vi "Tracepoint_LoadStaleFiles.vi"(8 "error in (no error)":errorcluster, 10 "file paths":path[](array[path]), 11 "Qbus in":refnum<class "Qbus.lvclass">) -> (0 "error out":errorcluster)   [LabVIEW 2017, in "FileManager.lvlib"]
uses:
  <vilib>/addons/InsightCM/Devices/Shared/Common/FileManager/FileManager.lvlib
  <vilib>/addons/Qbus/Qbus.lvclass
  <vilib>/addons/TraceLogger/TraceLogger.lvlib
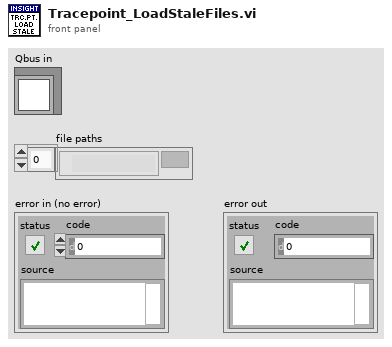
[diagram p1: front panel]
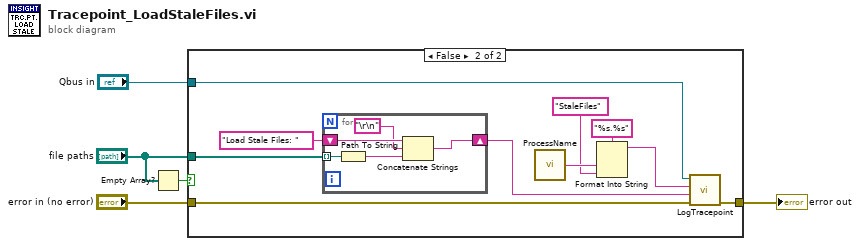
[diagram p0: block diagram]
diagram:
  n1 = Empty Array?(array="file paths") -> (empty?=w3:bool)
  n2 = case shown="False" w3 {
    tunnel: "file paths" -> [_ w9]
    tunnel: "error in (no error)" -> [w6 w12]
    tunnel: [w6 w11] -> w4
    tunnel: "Qbus in" -> [_ w10]
    frame True {
    }
    frame False {
      n3 = for {
        tunnel: w9 -> [w19] mode=indexing
        shift-right: [w21] -> w8
        shift-left: "Load Stale Files: " -> [w20]
        n4 = Path To String(path=w19) -> (string=w18:string)
        n5 = Concatenate Strings(w20, "\r\n", w18) -> (w21:string)
      }
      n6 = call <vilib>:"ProcessName.vi"() -> ("process name"=w16:string)  [unwired: 5 in]
      n7 = Format Into String(format string="%s.%s", w16, "StaleFiles" ("tracepoint")) -> (resulting string=w13:string)  [unwired: 2 in, 1 out]
      n8 = call <vilib>:"LogTracepoint.vi"("error in (no error)"=w12, "log string"=w8, "tracepoint"=w13, "qbus in"=w10) -> ("error out"=w11:errorcluster)  [unwired: 6 in, 1 out]
    }
  }
  "error out" <- w4
